vi "GetDiagramData.vi"(0 "reference":refnum<class "StateDiagramGraph.lvclass">, 5 "error in (no error)":errorcluster) -> (14 "reference out":refnum<class "StateDiagramGraph.lvclass">, 15 "DiagramData":string, 19 "error out":errorcluster)   [LabVIEW 2014, in "StateDiagramGraph.lvclass"]
doc: "GetDiagramData"
uses:
  <resource>/Framework/Providers/Open_GDS/UML/StateDiagramGraph_class/StateDiagramGraph.lvclass
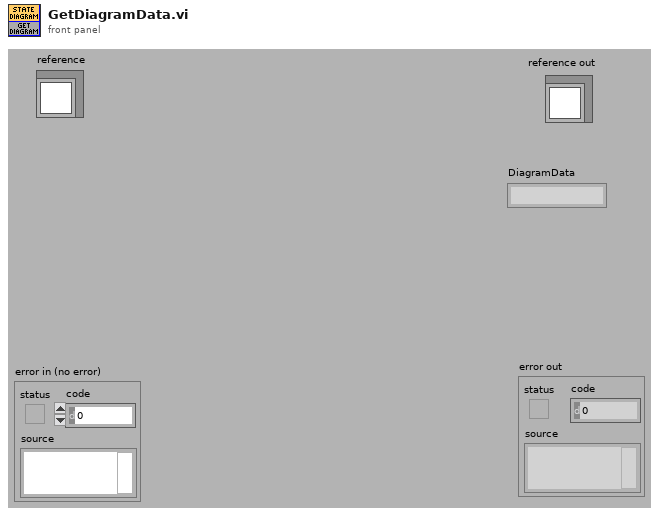
[diagram p1: front panel]
types:
  T1 = typedef "StateDiagramGraph.lvclass/ObjectAttributes.ctl" = cluster{"Base class":T2, "StateDiagramData":T3}
  T2 = typedef "Graph.lvclass/ObjectAttributes.ctl" = cluster{"nodes":refnum<class "AbstractNode.lvclass">[], "edges":refnum<class "AbstractEdge.lvclass">[], "nodesToBeRemoved":refnum<class "AbstractNode.lvclass">[], "edgesToBeRemoved":refnum<class "AbstractEdge.lvclass">[], "needsLayout":bool, "LayoutNodes":refnum<class "AbstractNode.lvclass">[]}
  T3 = typedef "StateDiagramGraph.lvclass/StateDiagramData.ctl" = cluster{"VI-Path":path, "ShowOption":T4}
  T4 = typedef "StateDiagramGraph.lvclass/ViPathShowOption.ctl" = enum16{"Don't Show", "Show Relative Path", "Show Absolute Path"}
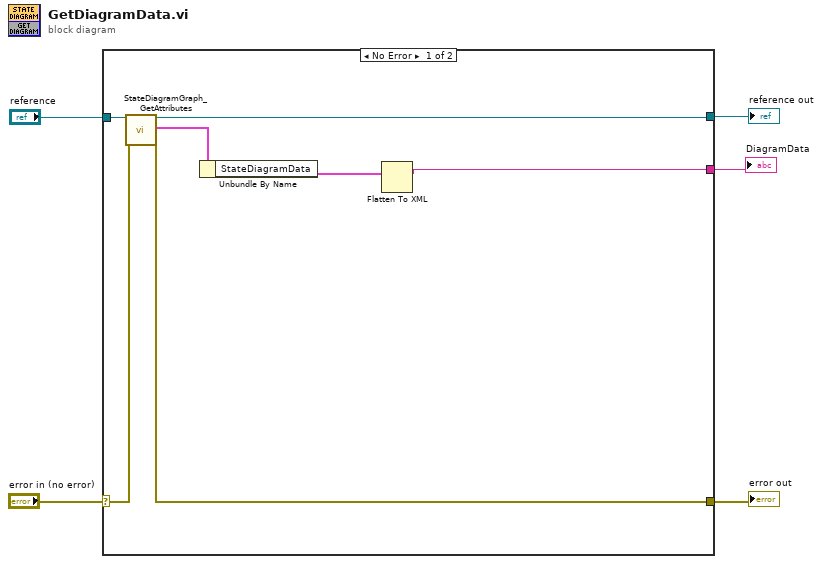
[diagram p0: block diagram]
diagram:
  n1 = case shown="No Error" "error in (no error)" {
    selector: "error in (no error)" -> [w12 w13]
    tunnel: "reference" -> [w11 w14]
    tunnel: [w8 w13] -> w3
    tunnel: [w9 w14] -> w2
    tunnel: [w6 _] -> w1
    frame No Error {
      n2 = call <resource>:"StateDiagramGraph_GetAttributes.vi"("reference in"=w11, "error in (no error)"=w12) -> ("reference out"=w9:refnum<class "StateDiagramGraph.lvclass">, "Attributes"=w10:T1, "error out"=w8:errorcluster)  [unwired: 15 out]
      n3 = Unbundle By Name(w10) -> ("StateDiagramData"=w7:T3)
      n4 = Flatten To XML(anything=w7) -> (xml string=w6:string)
    }
    frame Error {
    }
  }
  "reference out" <- w2
  "error out" <- w3
  "DiagramData" <- w1
